vi "LVClass_ModalCoef ctor from Subtract.vi"(0 "ModalCoef (const)":refnum<class "ModalCoef.lvclass">, 5 "ModalCoef A":refnum<class "ModalCoef.lvclass">, 7 "ModalCoef B":refnum<class "ModalCoef.lvclass">, 11 "error in (no error)":errorcluster) -> (4 "ModalCoef (new)":refnum<class "ModalCoef.lvclass">, 6 "ModalCoef A (dup)":refnum<class "ModalCoef.lvclass">, 8 "ModalCoef B (dup)":refnum<class "ModalCoef.lvclass">, 15 "error out":errorcluster)   [LabVIEW 2020, in "ModalCoef.lvclass"]
doc: "ModalCoef constructor.\n\n--------------------------------------------------------------------------------\n\n<B>ModalCoefIn </B> : Constant Pointer to ModalCoef object.\n<B>ModalCoefOut </B> : Constant Pointer to ModalCoef object.\n<B>TypePhase </B> : TypePhase Phase mode reconstruction.\n<B>ErrorIn </B> : Error\n<B>ErrorOut </B> : Error\n\n--------------------------------------------------------------------------------"
uses:
  ModalCoef.lvclass
  Controls/Handle creation.ctl
  ModalCoef.lvclass/ModalCoef.ctl
  LVClass_ModalCoef Read ModalCoef.vi
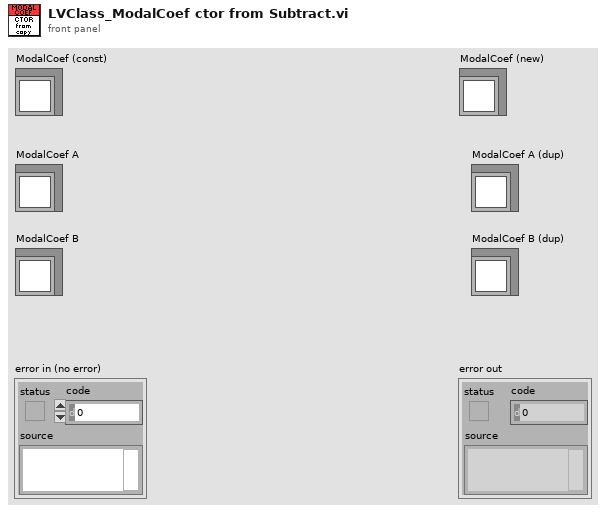
[diagram p1: front panel]
types:
  T1 = typedef "Handle creation.ctl" = enum16{"By ctor", "By write function"}
  T2 = typedef "ClassID.ctl" = i64
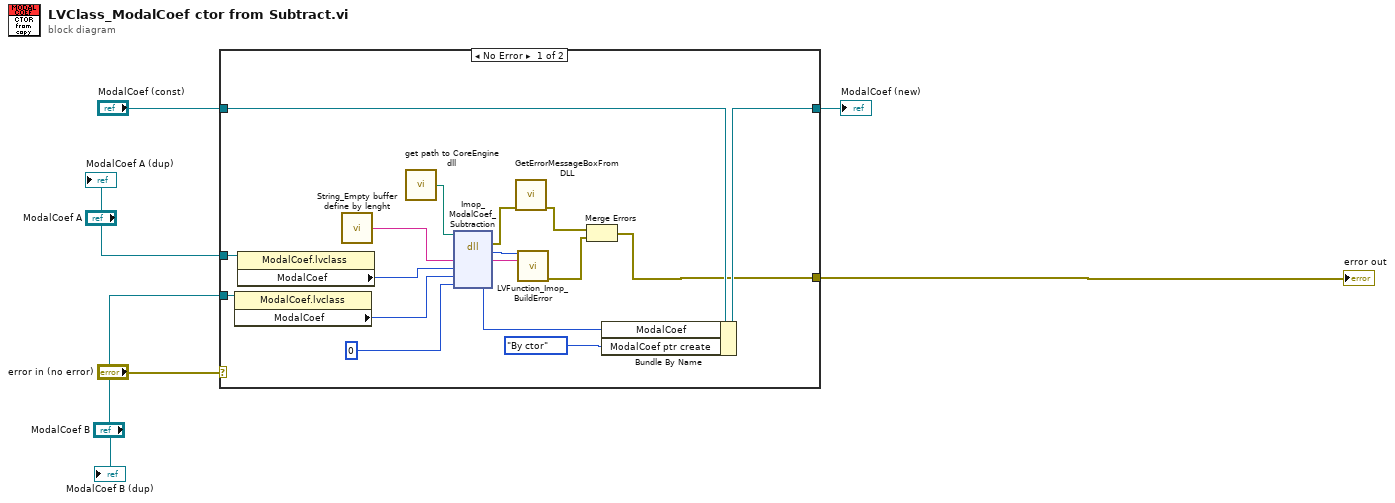
[diagram p0: block diagram]
diagram:
  n1 = case shown="No Error" "error in (no error)" {
    selector: "error in (no error)" -> [_ w25]
    tunnel: [w11 w25] -> w5
    tunnel: [w14 w24] -> w3
    tunnel: "ModalCoef (const)" -> [w15 w24]
    tunnel: "ModalCoef A" -> [w10 _]
    tunnel: "ModalCoef B" -> [w8 _]
    frame No Error {
      n2 = property class="ModalCoef.lvclass"(reference=w8) -> ("ModalCoef"=w7:T2)  [unwired: 1 in, 2 out]
      n3 = property class="ModalCoef.lvclass"(reference=w10) -> ("ModalCoef"=w9:T2)  [unwired: 1 in, 2 out]
      n4 = call "String_Empty buffer define by lenght.vi"() -> ("Empty buffer"=w23:string)  [unwired: 1 in]
      n5 = call "get path to CoreEngine dll.vi"() -> ("path to wavekit library"=w20:path)  [unwired: 14 in, 1 out]
      n6 = dll-call lib="D:/soft/HASO_v3/SVN_trunk/ImOpCoreEngine4_LV2011/DLLs/c_interface_vc100.dll" fn="Imop_ModalCoef_Subtraction"(path in=w20, "message"=w23, "ModalCoefA"=w9, "ModalCoefB"=w7, "ModalCoef"=0 ("Pupil")) -> (error out=w19:errorcluster, "return type"=w21:i32, "message"=w22:string, "ModalCoef"=w17:i64)  [unwired: 4 in, 1 out]
      n7 = call "GetErrorMessageBoxFromDLL.vi"("error IN"=w19) -> ("error OUT"=w13:errorcluster)  [unwired: 10 in]
      n8 = call "LVFunction_Imop_BuildError.vi"("code"=w21, "String to Prepend to source (\"\")"=w22) -> ("error out"=w12:errorcluster)  [unwired: 13 in]
      n9 = Merge Errors(w13, w12) -> (w11:errorcluster)
      n10 = Bundle By Name(cluster=w15, "ModalCoef"=w17, "ModalCoef ptr create"=Handle_creation."By ctor" ("Pupil ptr create")) -> (w14:refnum<class "ModalCoef.lvclass">)
    }
    frame Error {
    }
  }
  "error out" <- w5
  "ModalCoef (new)" <- w3
  "ModalCoef A (dup)" <- "ModalCoef A"
  "ModalCoef B (dup)" <- "ModalCoef B"
